vi "re_VI.execute_lua.vi"(5 "LuaVIEW reference":T1) -> (15 "error out":errorcluster)   [LabVIEW 2012]
doc: "Executes a VI synchronously. This method maps to the LabVIEW run VI method with the \"Wait until done\" option set so that it does not return until the VI completes execution.\nParameters:\nobj:self, object of VI to execute.\nErrors:\nNot a VI object.\nDead VI object.\nCould not execute VI."
uses:
  typedefs/t_LuaVIEW Reference.ctl
  subvis/private/LuaVIEW Pull (object).vi
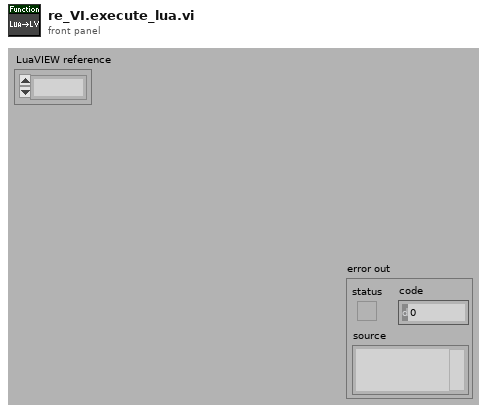
[diagram p1: front panel]
types:
  T1 = typedef "t_LuaVIEW Reference.ctl" = refnum<k1>
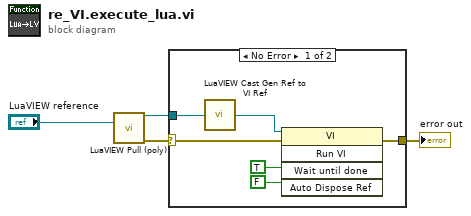
[diagram p0: block diagram]
diagram:
  n1 = call-poly "LuaVIEW Pull (poly).vi"("LuaVIEW reference in"="LuaVIEW reference") -> ("object refnum"=w2:refnum<vi>, "error out"=w1:errorcluster)  [unwired: 11 in, 2 out]
  n2 = case shown="No Error" w1 {
    selector: w1 -> [w10 w11]
    tunnel: [w8 w11] -> w3
    tunnel: w2 -> [w6 _]
    frame No Error {
      n3 = call "LuaVIEW Cast Gen Ref to VI Ref.vi"("refnum in"=w6) -> ("refnum out"=w9:refnum<vi>)  [unwired: 14 in]
      n4 = invoke class="VI" method="Run VI"(reference=w9, error in=w10, "Wait until done"=TRUE, "Auto Dispose Ref"=FALSE) -> (error out=w8:errorcluster)  [unwired: 1 in, 4 out]
    }
    frame Error {
    }
  }
  "error out" <- w3
